vi "LimitesTable.vi"(2 "error in":errorcluster, 3 "PNGs in folder":string[](array[string]), 4 "Folder path":path) -> (0 "error out":errorcluster, 1 "Billard rect":T2)   [LabVIEW 2025]
panel:
  out "B":u8
  out "G":u8
  out "R":u8
  in  "Final":T1
  out "X":i32
  out "Y":i32
  in  "Dark blue frame":T3={"Rmax"=24, "Rmin "=0, "Gmax"=49, "Gmin"=0, "Bmax"=119, "Bmin "=100}
  in  "Initial":T1
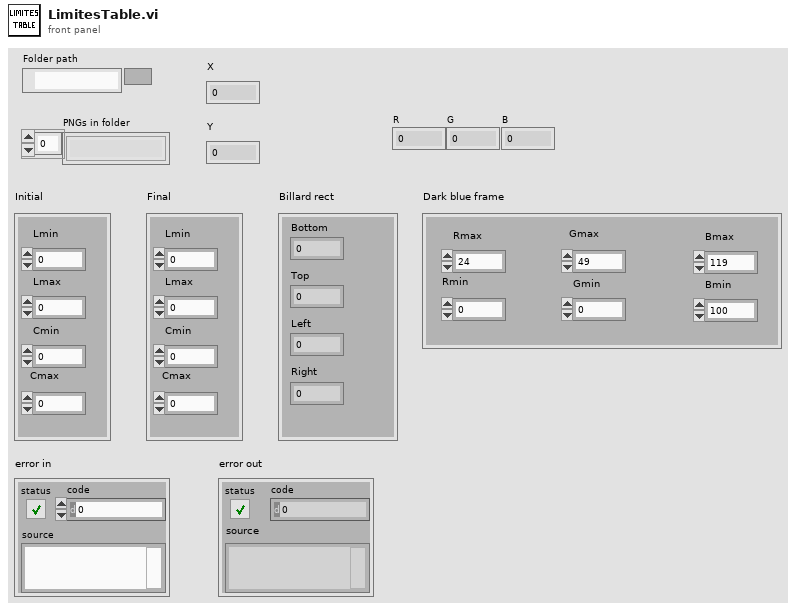
[diagram p1: front panel]
types:
  T1 = cluster{"Lmin":i32, "Lmax ":i32, "Cmin":i32, "Cmax":i32}
  T2 = cluster{"Bottom":dbl, "Top":dbl, "Left":dbl, "Right":dbl}
  T3 = cluster{"Rmax":i32, "Rmin ":i32, "Gmax":i32, "Gmin":i32, "Bmax":i32, "Bmin ":i32}
  T4 = typedef "imagedata.ctl" = cluster{"image type":i32, "image depth":i32, "image":u8[], "mask":u8[], "colors":u32[], "Rectangle":cluster{"left":i16, "top":i16, "right":i16, "bottom":i16}}
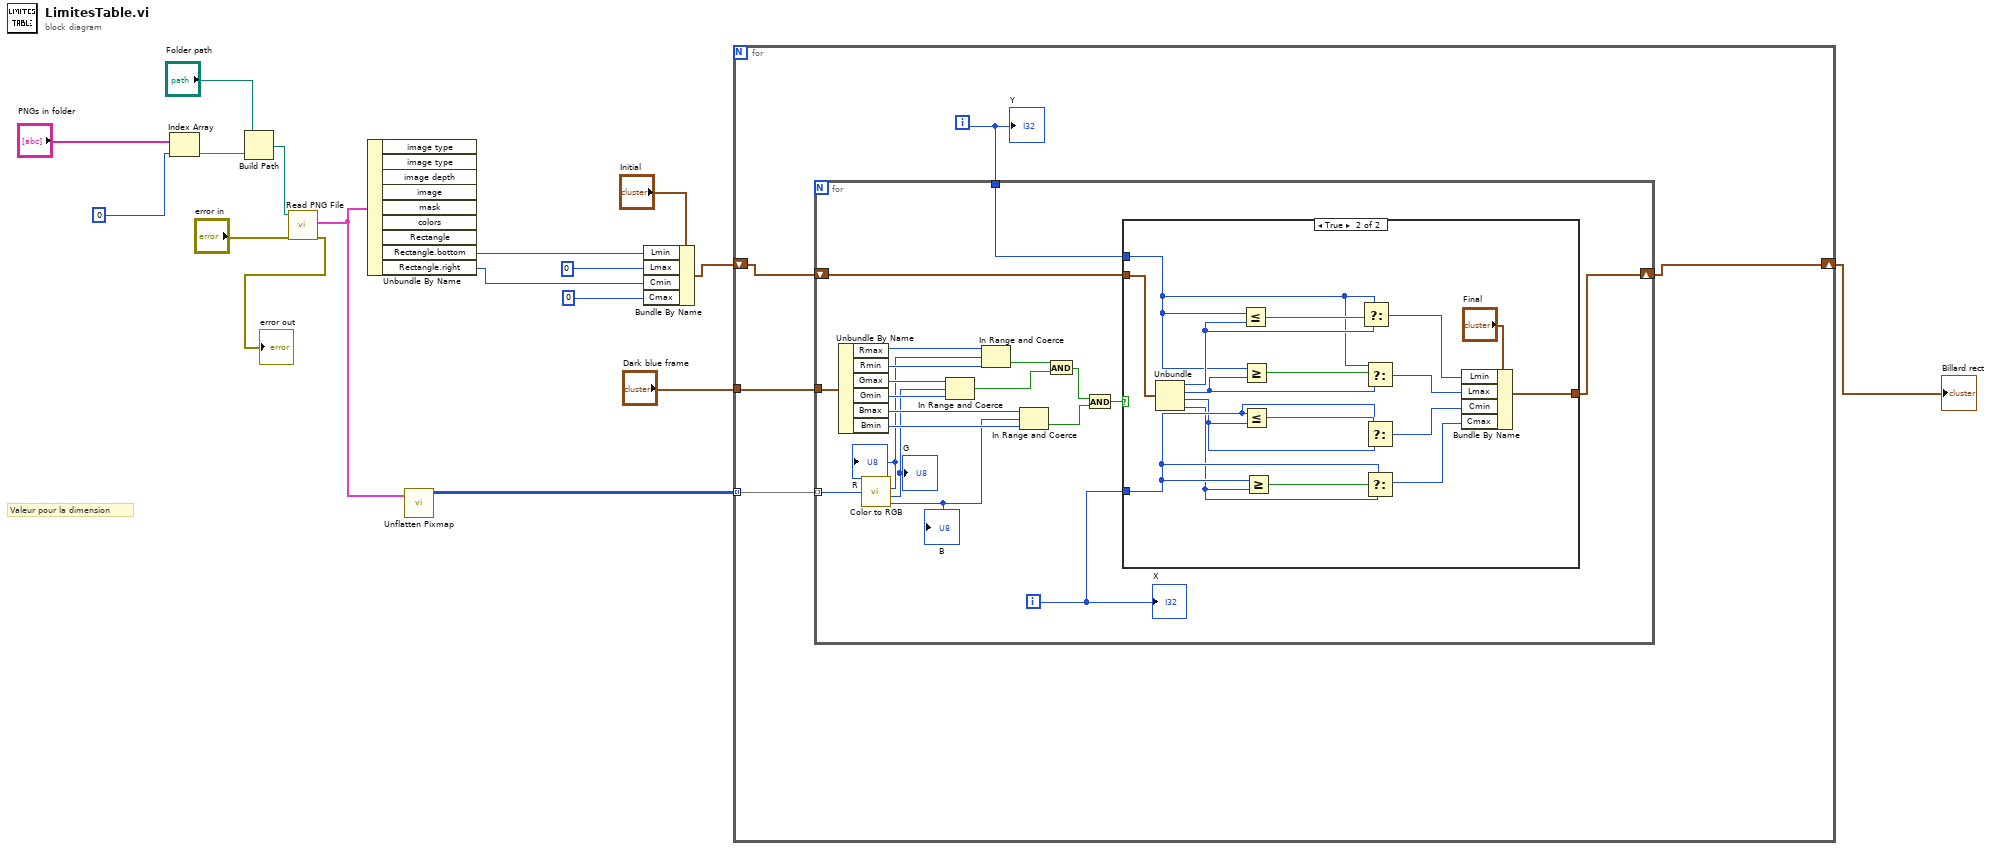
[diagram p0: block diagram]
diagram:
  # "Valeur pour la dimension"
  n1 = Index Array(array="PNGs in folder", index=0) -> (element=w15:string)
  n2 = Build Path(base path="Folder path", name or relative path=w15) -> (appended path=w14:path)
  n3 = call <vilib>:"Read PNG File.vi"("error in (no error)"="error in", "path to PNG file"=w14) -> ("error out"=→"error out":errorcluster, "image data"=w13:T4)  [unwired: 7 in, 1 out]
  n4 = Unbundle By Name(w13) -> ("Rectangle.bottom"=w5:i16, "Rectangle.right"=w4:i16)  [unwired: 7 out]
  n5 = call <vilib>:"Unflatten Pixmap.vi"("image data"=w13) -> ("24-bit pixmap"=w10:u32[][])  [unwired: 4 in, 6 out]
  n6 = Bundle By Name(cluster="Initial", "Lmin"=w5, "Lmax"=0, "Cmin"=w4, "Cmax"=0) -> (w3:T1)
  n7 = for {
    tunnel: "Dark blue frame" -> [w22]
    tunnel: w10 -> [w21] mode=indexing
    shift-right: [w18] -> w2
    shift-left: w3 -> [w19]
    i -> [w20]
    n8 = for {
      tunnel: w22 -> [w42]
      tunnel: w21 -> [w41] mode=indexing
      tunnel: w20 -> [w29]
      shift-right: [w26] -> w18
      shift-left: w19 -> [w27]
      i -> [w28]
      n9 = Unbundle By Name(w42) -> ("Rmax"=w40:i32, "Rmin"=w39:i32, "Gmax"=w38:i32, "Gmin"=w37:i32, "Bmax"=w36:i32, "Bmin"=w35:i32)
      n10 = call <vilib>:"Color to RGB.vi"("Color"=w41) -> ("R"=w25:u8, "G"=w24:u8, "B"=w23:u8)  [unwired: 1 out]
      "R" <- w25
      "G" <- w24
      "B" <- w23
      n11 = In Range and Coerce(upper limit=w38, x=w24, lower limit=w37) -> (In Range?=w33:bool)  [unwired: 1 out]
      n12 = In Range and Coerce(upper limit=w40, x=w25, lower limit=w39) -> (In Range?=w34:bool)  [unwired: 1 out]
      n13 = In Range and Coerce(upper limit=w36, x=w23, lower limit=w35) -> (In Range?=w31:bool)  [unwired: 1 out]
      n14 = And(x=w34, y=w33) -> (x .and. y?=w32:bool)
      n15 = And(x=w32, y=w31) -> (x .and. y?=w30:bool)
      n16 = case shown="True" w30 {
        tunnel: w27 -> [w43 w60]
        tunnel: w29 -> [_ w51]
        tunnel: w28 -> [_ w49]
        tunnel: [w43 w46] -> w26
        frame False {
        }
        frame True {
          n17 = Unbundle(w60) -> ("Lmin"=w52:i32, "Lmax"=w50:i32, "Cmin"=w47:i32, "Cmax"=w48:i32)
          n18 = Less Or Equal?(x=w51, y=w52) -> (x <= y?=w59:bool)
          n19 = Greater Or Equal?(x=w51, y=w50) -> (x >= y?=w58:bool)
          n20 = Less Or Equal?(x=w49, y=w47) -> (x <= y?=w57:bool)
          n21 = Greater Or Equal?(x=w49, y=w48) -> (x >= y?=w56:bool)
          n22 = Select(t=w51, s=w59, f=w52) -> (s? t:f=w44:i32)
          n23 = Select(t=w51, s=w58, f=w50) -> (s? t:f=w55:i32)
          n24 = Select(t=w49, s=w57, f=w47) -> (s? t:f=w54:i32)
          n25 = Select(t=w49, s=w56, f=w48) -> (s? t:f=w53:i32)
          n26 = Bundle By Name(cluster="Final", "Lmin"=w44, "Lmax"=w55, "Cmin"=w54, "Cmax"=w53) -> (w46:T1)
        }
      }
      "X" <- w28
    }
    "Y" <- w20
  }
  "Billard rect" <- w2
